vi "random dice.vi"(0 "Player1 roll":bool, 1 "dice1 state":u8, 5 "button1 state":bool, 9 "Player2 roll":bool, 11 "button2 state":bool, 12 "dice2 state":u8) -> (2 "Player1 Finish":bool, 3 "button1 next_state":bool, 4 "Player1 Dice":u8, 6 "Player2 Dice":u8, 10 "Dice rolling instr.":string, 13 "Player2 Finish":bool, 14 "button2 next_state":bool, 15 "both finished":bool)   [LabVIEW 2014]
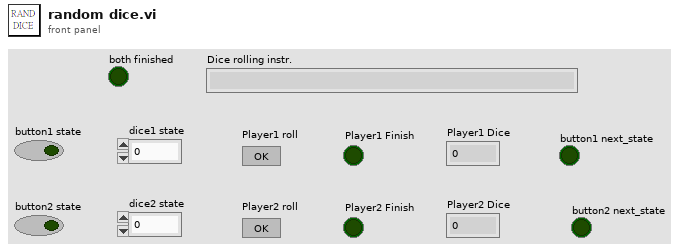
[diagram p1: front panel]
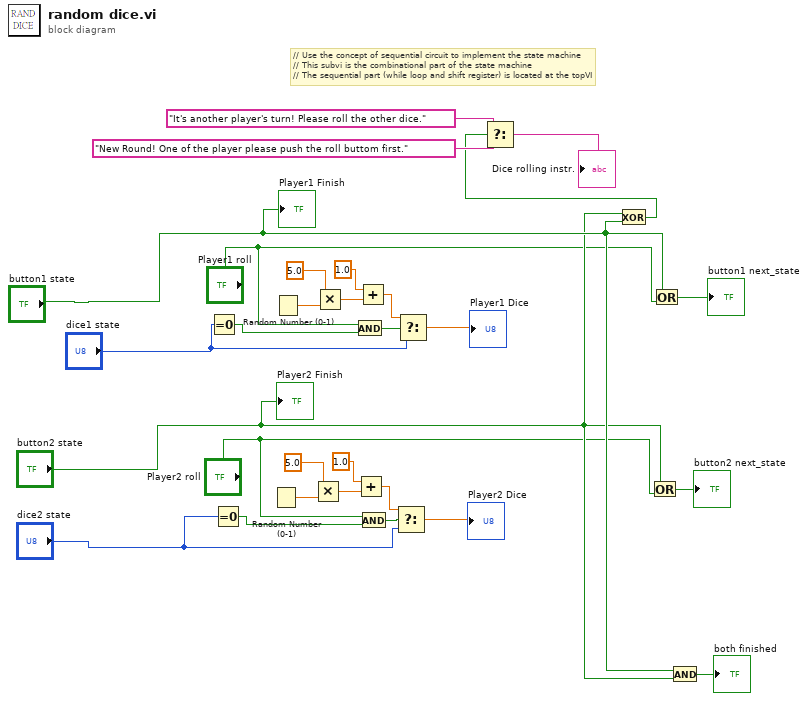
[diagram p0: block diagram]
diagram:
  # "// Use the concept of sequential circuit to implement the state machine\n// This subvi is the combinational part of the state machine\n// The sequential part (while loop and shift register) is located at the topVI"
  n1 = Equal To 0?(x="dice1 state") -> (x = 0?=w11:bool)
  n2 = Equal To 0?(x="dice2 state") -> (x = 0?=w10:bool)
  n3 = Random Number (0-1)() -> (number: 0 to 1=w18:dbl)
  n4 = Random Number (0-1)() -> (number: 0 to 1=w24:dbl)
  n5 = Multiply(x=5.0, y=w18) -> (x*y=w17:dbl)
  n6 = Multiply(x=5.0, y=w24) -> (x*y=w23:dbl)
  n7 = And(x="Player1 roll", y=w11) -> (x .and. y?=w13:bool)
  n8 = Add(x=1.0, y=w17) -> (x+y=w15:dbl)
  n9 = Add(x=1.0, y=w23) -> (x+y=w21:dbl)
  n10 = And(x="Player2 roll", y=w10) -> (x .and. y?=w9:bool)
  n11 = Select(t=w15, s=w9, f="dice2 state") -> (s? t:f=→"Player2 Dice":dbl)
  n12 = Select(t=w21, s=w13, f="dice1 state") -> (s? t:f=→"Player1 Dice":dbl)
  n13 = Exclusive Or(1:"button1 state", 2:"button2 state") -> (0:w4:bool)
  n14 = Select(t="It's another player's turn! Please roll the other dice." ("f"), s=w4, f="New Round! One of the player please push the roll buttom first." ("t")) -> (s? t:f=→"Dice rolling instr.":string)
  n15 = Or(x="button2 state", y="Player2 roll") -> (x .or. y?=→"button2 next_state":bool)
  n16 = Or(x="button1 state", y="Player1 roll") -> (x .or. y?=→"button1 next_state":bool)
  n17 = And(x="button1 state", y="button2 state") -> (x .and. y?=→"both finished":bool)
  "Player1 Finish" <- "button1 state"
  "Player2 Finish" <- "button2 state"
